vi "IV_curve_measurement_PO.vi"(9 "Channel":T1, 11 "VISA resource name":refnum<visa-resource-name>="GPIB0::26::INSTR") -> ()   [LabVIEW 2009]
doc: "This example shows how to configure the source and take a measurement."
uses:
  <instrlib>/Keithley 2600 Series/Public/Channel.ctl
  <vilib>/express/express signal manip/GetorSetDDTAttributes/Set DDT Attributes/Set DDT Properties.xnode
  <vilib>/express/express shared/transition.llb/Waveform Array To Dynamic.vi
  <vilib>/express/express signal manip/GetorSetDDTAttributes/Set DDT Attributes/SetT0.vi
  <vilib>/express/express shared/transition.llb/Dynamic To Waveform Array.vi
  <instrlib>/Keithley 2600 Series/Keithley 2600 Series.lvlib
panel:
  in  "Tab Control":enum32{"Measurement", "Control Panel"}(tab)
  in  "Current Limit (A)":dbl
  in  "Plot Set/Meas voltage":bool
  out "PV - Curve":cluster{"Y":dbl[], "Y":dbl[]}[](graph)
  in  "Post output":bool caption="POST output"
  in  "Post Currrent limit (A)":dbl=0.1
  out "IV - Curve":cluster{"Y":dbl[], "Y":dbl[]}[](graph)
  in  "Number of points":dbl=300.0
  in  "Start voltage (V)":dbl=-1.0
  in  "End voltage (V)":dbl=1.0
  in  "Delay between points (ms)":u32=10
  out "dV (V)":dbl=0.006666666666666667
  out "Set Voltage point (V)":dbl=1.500000000000001
  out "Current point (A)":dbl=-7.54118e-11
  out "Differential resistance (Ohm)":dbl
  out "Mean resistance (Ohm)":dbl
  in  "Post Voltage (V)":dbl=0.1
  in  "Sense (2 Wire)":enum32{"2 Wire", "4 Wire", "Calibration"}(ring)
  # "You have to press local on the instrument to show the measurement after the sweep"
  # "Power - Voltage Curve to see at what power the mesa dies"
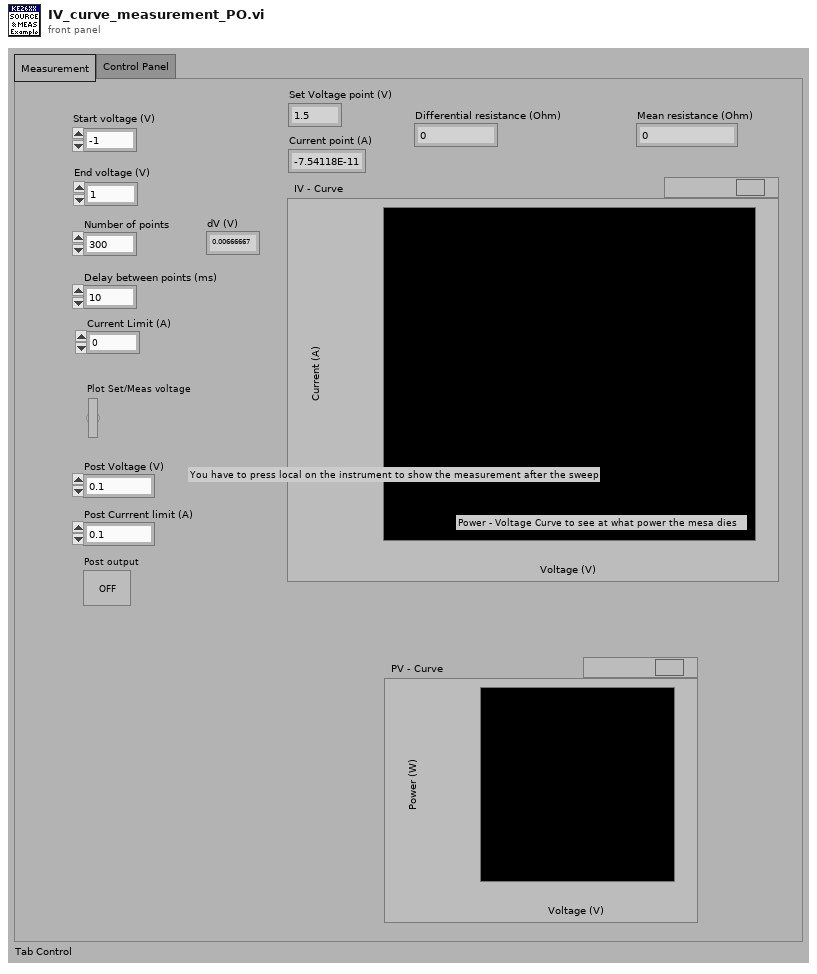
[diagram p1: front panel]
types:
  T1 = typedef "Keithley 2600 Series.lvlib/Channel.ctl" = enum32{"Channel A", "Channel B"}
  T2 = enum32{"Current", "Voltage", "IV", "Resistance", "Power"}
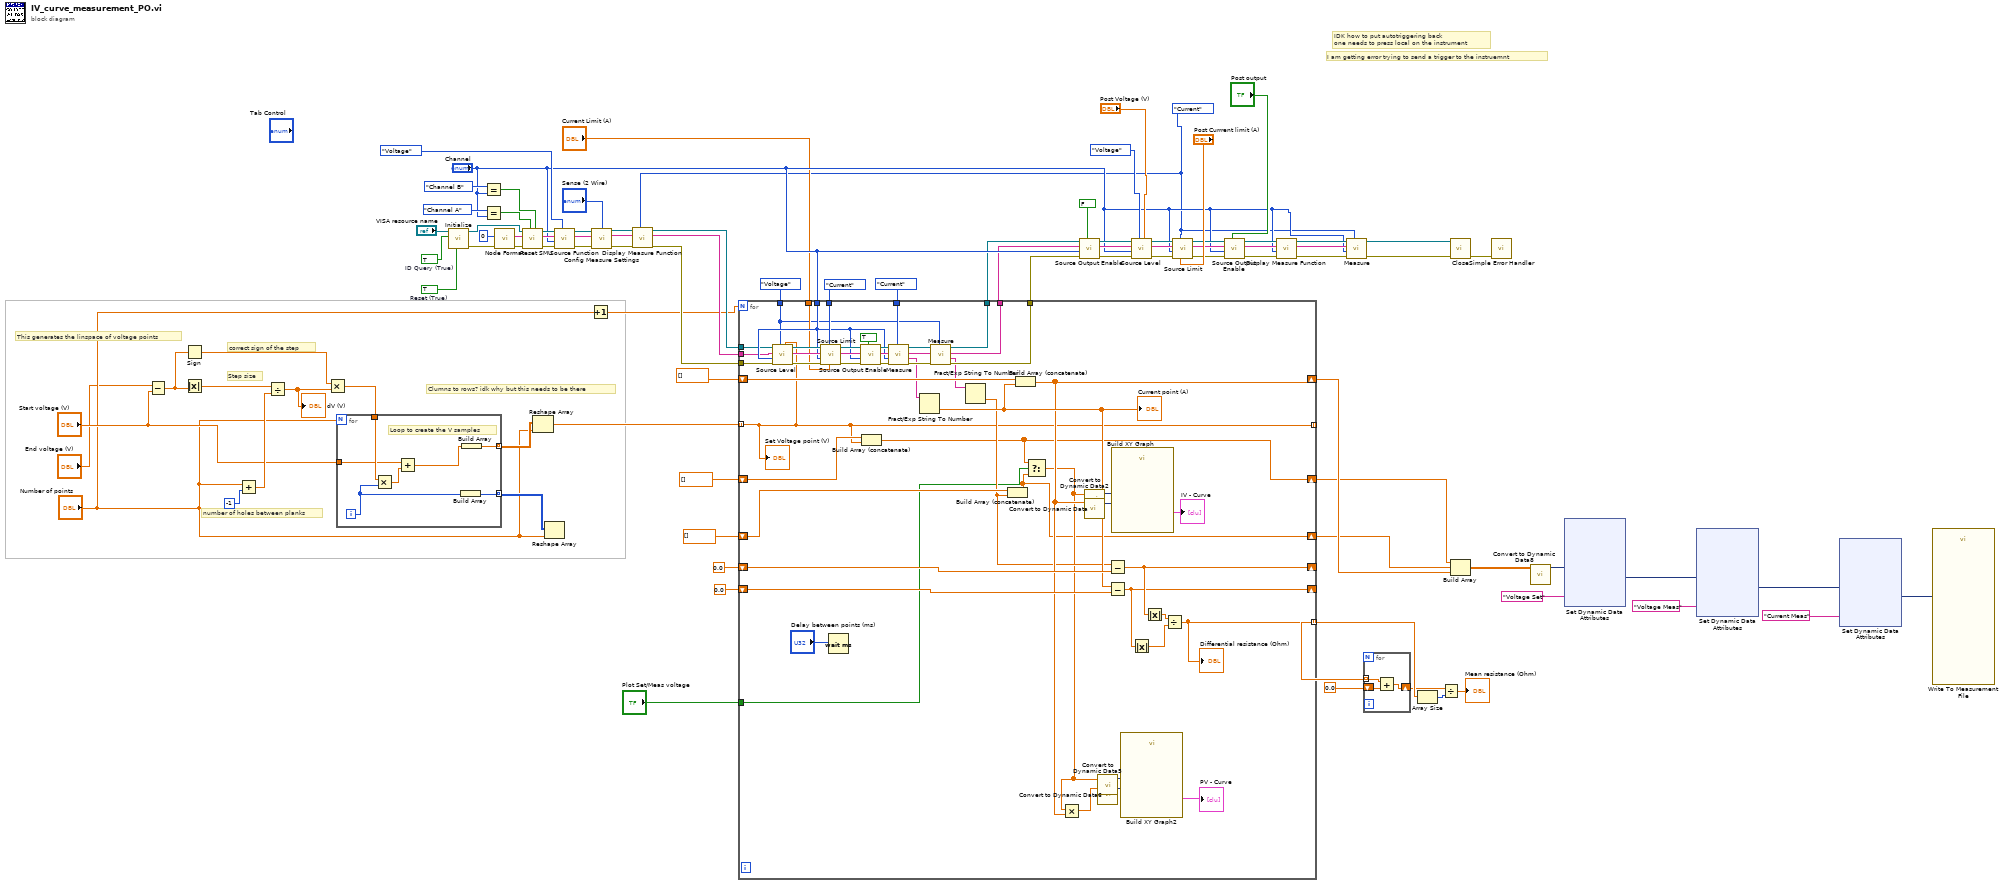
[diagram p0: block diagram]
diagram:
  w5 = enum32{"Current", "Voltage"}."Current" ("Function (Current)")
  w83 = TRUE  # Reset (True)
  w93 = TRUE  # ID Query (True)
  # "This generates the linspace of voltage points"
  # "I am getting error trying to send a trigger to the instruemnt"
  # "IDK how to put autotriggering back\none needs to press local on the instrument"
  # "Clumns to rows? idk why but this needs to be there"
  # "number of holes between planks"
  # "correct sign of the step"
  # "Step size"
  n1 = Subtract(x="End voltage (V)", y="Start voltage (V)") -> (x-y=w59:dbl)
  n2 = Sign(1:w59) -> (0:w58:dbl)
  n3 = Absolute Value(x=w59) -> (abs(x)=w53:dbl)
  n4 = Add(x="Number of points", y=-1) -> (x+y=w63:dbl)
  n5 = Divide(x=w53, y=w63) -> (x/y=w38:dbl)
  "dV (V)" <- w38
  n6 = Multiply(x=w58, y=w38) -> (x*y=w57:dbl)
  n7 = for {
    N: "Number of points" -> [_]
    tunnel: w57 -> [w101]
    tunnel: "Start voltage (V)" -> [w99]
    tunnel: [w97] -> w61 mode=indexing
    tunnel: [w95] -> w60 mode=indexing
    i -> [w96]
    # "Loop to create the V samples"
    n8 = Multiply(x=w101, y=w96) -> (x*y=w100:dbl)
    n9 = Add(x=w99, y=w100) -> (x+y=w98:dbl)
    n10 = Build Array(w96) -> (w95:i32[])
    n11 = Build Array(w98) -> (w97:dbl[])
  }
  n12 = call <instrlib>:"Initialize.vi"("Reset (True)"=w83, "ID Query (True)"=w93, "VISA resource name"="VISA resource name") -> ("error out"=w81:errorcluster, "VISA resource name out"=w92:refnum<visa-resource-name>)  [unwired: 3 in, 4 out]
  n13 = Equal?(x=enum32{"Channel A", "Channel B"}."Channel B", y="Channel") -> (x = y?=w88:bool)
  n14 = Equal?(x=enum32{"Channel A", "Channel B"}."Channel A", y="Channel") -> (x = y?=w89:bool)
  n15 = call <instrlib>:"Node Format.vi"("error in"=w81, "Node (0-64)"=i8 0) -> ("error out"=w80:errorcluster, "Formatted Node"=w82:string)  [unwired: 8 out]
  n16 = call <instrlib>:"Reset SMU.vi"("SMU B (No)"=w88, "SMU A (No)"=w89, "error in (no error)"=w80, "Node In"=w82, "VISA resource name"=w92) -> ("error out"=w87:errorcluster, "Node Out"=w85:string, "VISA resource name out"=w86:refnum<visa-resource-name>)  [unwired: 4 out]
  n17 = Reshape Array(w61, "Number of points") -> (w56:dbl[])
  n18 = Reshape Array(w60, "Number of points") -> ()  [unwired: 1 out]
  n19 = call <instrlib>:"Source Function.vi"("Function (Current)"=enum32{"Current", "Voltage"}."Voltage", "error in (no error)"=w87, "Channel (Channel A)"="Channel", "Node In"=w85, "VISA resource name"=w86) -> ("error out"=w65:errorcluster, "Node Out"=w9:string, "VISA resource name out"=w10:refnum<visa-resource-name>)  [unwired: 4 out]
  n20 = Increment(x="Number of points") -> (x+1=w1:dbl)
  n21 = call <instrlib>:"Config Measure Settings.vi"("VISA resource name"=w10, "Sense (2 Wire)"="Sense (2 Wire)", "Node In"=w9, "error in"=w65) -> ("VISA resource name out"=w6:refnum<visa-resource-name>, "Node Out"=w7:string, "error out"=w8:errorcluster)  [unwired: 8 in, 1 out]
  n22 = call <instrlib>:"Display Measure Function.vi"("Function (Current)"=w5, "error in (no error)"=w8, "Node In"=w7, "VISA resource name"=w6) -> ("error out"=w2:errorcluster, "Node Out"=w3:string, "VISA resource name out"=w4:refnum<visa-resource-name>)  [unwired: 4 in, 1 out]
  n23 = for {
    N: w1 -> [_]
    tunnel: "Channel" -> [w129]
    shift-right: [w126] -> w23
    shift-left: dbl[] [] -> [w142]
    shift-right: [w113] -> w22
    shift-left: dbl[] [] -> [w140]
    tunnel: enum32{"Current", "Voltage"}."Voltage" ("Function (Current)") -> [w109]
    tunnel: enum32{"Current", "Voltage"}."Current" ("Function (Current)") -> [w137]
    tunnel: T2."Current" ("Function (Current)") -> [w136]
    shift-right: [w132] -> _
    shift-left: 0.0 -> [w135]
    shift-right: [w131] -> _
    shift-left: 0.0 -> [w133]
    tunnel: [w130] -> w70 mode=indexing
    tunnel: w56 -> [w115] mode=indexing
    tunnel: [w115] -> _ mode=indexing
    tunnel: [w120] -> w27
    tunnel: [w119] -> w26
    tunnel: [w118] -> w25
    shift-right: [w112] -> w21
    shift-left: dbl[] [] -> [w116]
    tunnel: "Plot Set/Meas voltage" -> [w111]
    tunnel: "Current Limit (A)" -> [w110]
    tunnel: w4 -> [w108]
    tunnel: w3 -> [w107]
    tunnel: w2 -> [w106]
    n24 = call <instrlib>:"Source Level.vi"("Level (0.000)"=w115, "Function (Current)"=w109, "error in (no error)"=w106, "Channel (Channel A)"=w129, "Node In"=w107, "VISA resource name"=w108) -> ("error out"=w153:errorcluster, "Node Out"=w146:string, "VISA resource name out"=w152:refnum<visa-resource-name>)  [unwired: 3 out]
    n25 = call <instrlib>:"Source Limit.vi"("Limit (0.000)"=w110, "Function (Current)"=w137, "error in (no error)"=w153, "Channel (Channel A)"=w129, "Node In"=w146, "VISA resource name"=w152) -> ("error out"=w150:errorcluster, "Node Out"=w145:string, "VISA resource name out"=w151:refnum<visa-resource-name>)  [unwired: 3 out]
    n26 = Wait (ms)(milliseconds to wait="Delay between points (ms)") -> ()  [unwired: 1 out]
    n27 = call <instrlib>:"Source Output Enable.vi"("Output (Off)"=TRUE, "error in (no error)"=w150, "Channel (Channel A)"=w129, "Node In"=w145, "VISA resource name"=w151) -> ("error out"=w149:errorcluster, "Node Out"=w144:string, "VISA resource name out"=w148:refnum<visa-resource-name>)  [unwired: 4 out]
    n28 = Build Array (concatenate)(w116, w115) -> (w112:dbl[])
    n29 = call <instrlib>:"Measure.vi"("Function (Current)"=w136, "error in (no error)"=w149, "Channel (Channel A)"=w129, "Node In"=w144, "VISA resource name"=w148) -> ("error out"=w123:errorcluster, "Output"=w105:string, "Node Out"=w122:string, "VISA resource name out"=w121:refnum<visa-resource-name>)  [unwired: 2 in, 1 out]
    n30 = Fract/Exp String To Number(string=w105) -> (number=w134:dbl)  [unwired: 3 in, 1 out]
    "Current point (A)" <- w134
    n31 = call <instrlib>:"Measure.vi"("Function (Current)"=w109, "error in (no error)"=w123, "Node In"=w122, "VISA resource name"=w121) -> ("error out"=w118:errorcluster, "Output"=w104:string, "Node Out"=w119:string, "VISA resource name out"=w120:refnum<visa-resource-name>)  [unwired: 3 in, 1 out]
    n32 = Fract/Exp String To Number(string=w104) -> (number=w117:dbl)  [unwired: 3 in, 1 out]
    n33 = Build Array (concatenate)(w140, w117) -> (w113:dbl[])
    n34 = Build Array (concatenate)(w142, w134) -> (w126:dbl[])
    n35 = Select(t=w112, s=w111, f=w113) -> (s? t:f=w114:dbl[])
    n36 = Multiply(x=w114, y=w126) -> (x*y=w125:dbl[])
    n37 = call "Convert to Dynamic Data"("Array"=w126) -> ("Dynamic Data Type"=w141:dynamicdata)  [unwired: 3 in]
    n38 = call "Convert to Dynamic Data2"("Array"=w114) -> ("Dynamic Data Type"=w139:dynamicdata)  [unwired: 3 in]
    n39 = call "Convert to Dynamic Data5"("Array"=w114) -> ("Dynamic Data Type"=w127:dynamicdata)  [unwired: 3 in]
    n40 = call "Convert to Dynamic Data6"("Array"=w125) -> ("Dynamic Data Type"=w124:dynamicdata)  [unwired: 3 in]
    n41 = Subtract(x=w117, y=w135) -> (x-y=w132:dbl)
    n42 = Subtract(x=w134, y=w133) -> (x-y=w131:dbl)
    n43 = call "Build XY Graph"("Y Input"=w141, "X Input"=w139) -> ("XY Graph"=→"IV - Curve":cluster{"Y":dbl[], "Y":dbl[]}[])  [unwired: 8 in, 1 out]
    n44 = call "Build XY Graph2"("Y Input"=w124, "X Input"=w127) -> ("XY Graph"=→"PV - Curve":cluster{"Y":dbl[], "Y":dbl[]}[])  [unwired: 8 in, 1 out]
    n45 = Absolute Value(x=w131) -> (abs(x)=w102:dbl)
    n46 = Absolute Value(x=w132) -> (abs(x)=w103:dbl)
    n47 = Divide(x=w103, y=w102) -> (x/y=w130:dbl)
    "Differential resistance (Ohm)" <- w130
    "Set Voltage point (V)" <- w115
  }
  n48 = call <instrlib>:"Source Output Enable.vi"("Output (Off)"=FALSE, "error in (no error)"=w25, "Channel (Channel A)"="Channel", "Node In"=w26, "VISA resource name"=w27) -> ("error out"=w51:errorcluster, "Node Out"=w49:string, "VISA resource name out"=w50:refnum<visa-resource-name>)  [unwired: 4 out]
  n49 = call <instrlib>:"Source Level.vi"("Level (0.000)"="Post Voltage (V)", "Function (Current)"=enum32{"Current", "Voltage"}."Voltage", "error in (no error)"=w51, "Channel (Channel A)"="Channel", "Node In"=w49, "VISA resource name"=w50) -> ("error out"=w46:errorcluster, "Node Out"=w45:string, "VISA resource name out"=w44:refnum<visa-resource-name>)  [unwired: 2 in, 1 out]
  n50 = call <instrlib>:"Source Limit.vi"("Limit (0.000)"="Post Currrent limit (A)", "Function (Current)"=w5, "error in (no error)"=w46, "Channel (Channel A)"="Channel", "Node In"=w45, "VISA resource name"=w44) -> ("error out"=w42:errorcluster, "Node Out"=w40:string, "VISA resource name out"=w41:refnum<visa-resource-name>)  [unwired: 3 out]
  n51 = call <instrlib>:"Source Output Enable.vi"("Output (Off)"="Post output", "error in (no error)"=w42, "Channel (Channel A)"="Channel", "Node In"=w40, "VISA resource name"=w41) -> ("error out"=w37:errorcluster, "Node Out"=w36:string, "VISA resource name out"=w35:refnum<visa-resource-name>)  [unwired: 4 out]
  n52 = call <instrlib>:"Display Measure Function.vi"("error in (no error)"=w37, "Channel (Channel A)"="Channel", "Node In"=w36, "VISA resource name"=w35) -> ("error out"=w34:errorcluster, "Node Out"=w32:string, "VISA resource name out"=w33:refnum<visa-resource-name>)  [unwired: 4 in, 1 out]
  n53 = call <instrlib>:"Measure.vi"("Function (Current)"=w5, "error in (no error)"=w34, "Channel (Channel A)"="Channel", "Node In"=w32, "VISA resource name"=w33) -> ("error out"=w29:errorcluster, "VISA resource name out"=w30:refnum<visa-resource-name>)  [unwired: 2 in, 3 out]
  n54 = for {
    tunnel: w70 -> [w156] mode=indexing
    shift-right: [w154] -> w68
    shift-left: 0.0 -> [w155]
    n55 = Add(x=w156, y=w155) -> (x+y=w154:dbl)
  }
  n56 = Array Size(array=w70) -> (size(s)=w69:i32)
  n57 = Divide(x=w68, y=w69) -> (x/y=→"Mean resistance (Ohm)":dbl)
  n58 = call <instrlib>:"Close.vi"("error in (no error)"=w29, "VISA resource name"=w30) -> ("error out"=w66:errorcluster)  [unwired: 9 out]
  n59 = Build Array(w21, w22, w23) -> (w18:dbl[][])
  n60 = call <vilib>:"Simple Error Handler.vi"("error in (no error)"=w66) -> ()  [unwired: 4 in, 5 out]
  n61 = call "Convert to Dynamic Data8"("2D Array"=w18) -> ("Dynamic Data Type"=w20:dynamicdata)  [unwired: 3 in]
  n62 = xnode "Set Dynamic Data Attributes"("Signals In"=w20, "Signal Name"="Voltage Set") -> ("Signals Out"=w17:dynamicdata)  [unwired: 2 in, 1 out]
  n63 = xnode "Set Dynamic Data Attributes"("Signals In"=w17, "Signal Name"="Voltage Meas") -> ("Signals Out"=w15:dynamicdata)  [unwired: 2 in, 1 out]
  n64 = xnode "Set Dynamic Data Attributes"("Signals In"=w15, "Signal Name"="Current Meas") -> ("Signals Out"=w14:dynamicdata)  [unwired: 2 in, 1 out]
  n65 = call "Write To Measurement File"("Signals"=w14) -> ()  [unwired: 16 in, 3 out]
